vi "Control_Create.vi"(7 "Object Attributes":T1, 8 "error in (no error)":errorcluster, 10 "Control Attributes":T3, 11 "Control In":refnum<class "Control.lvclass">) -> (0 "error out":errorcluster, 3 "Control Out":refnum<class "Control.lvclass">)   [LabVIEW 2015, in "Front Panel Publisher.lvlib" / "Control.lvclass"]
uses:
  Control.lvclass
  Attributes.ctl
  Text_class/Text.lvclass
  Object_class/Attributes.ctl
  Object_class/Coordinates.ctl
  Object_class/Object.lvclass
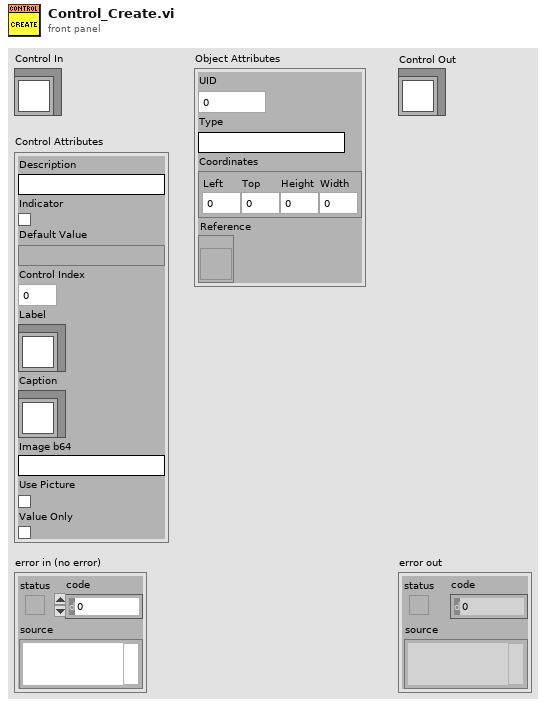
[diagram p1: front panel]
types:
  T1 = typedef "Front Panel Publisher.lvlib/Object.lvclass/Attributes.ctl" = cluster{"UID":i32, "Type":string, "Coordinates":T2, "Reference":refnum<vi>}
  T2 = typedef "Front Panel Publisher.lvlib/Object.lvclass/Coordinates.ctl" = cluster{"Left":i32, "Top":i32, "Height":u32, "Width":u32}
  T3 = typedef "Front Panel Publisher.lvlib/Control.lvclass/Attributes.ctl" = cluster{"Description":string, "Indicator":bool, "Default Value":variant, "Control Index":i32, "Label":refnum<class "Text.lvclass">, "Caption":refnum<class "Text.lvclass">, "Image b64":string, "Use Picture":bool, "Value Only":bool}
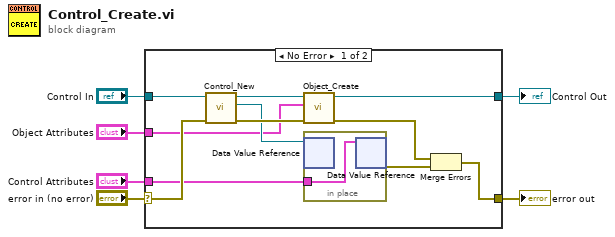
[diagram p0: block diagram]
diagram:
  n1 = case shown="No Error" "error in (no error)" {
    selector: "error in (no error)" -> [w16 w20]
    tunnel: [w14 w20] -> w5
    tunnel: "Control In" -> [w17 w19]
    tunnel: [w11 w19] -> w3
    tunnel: "Object Attributes" -> [w9 _]
    tunnel: "Control Attributes" -> [w8 _]
    frame No Error {
      n2 = call "Control_New.vi"("error in (no error)"=w16, "reference in"=w17) -> ("error out"=w12:errorcluster, "DVRRefOut"=w10:refnum<data-value>, "reference out"=w13:refnum<class "Control.lvclass">)  [unwired: 6 in, 1 out]
      n3 = call "Object_Create.vi"("error in (no error)"=w12, "Object Attributes"=w9, "Object In"=w13) -> ("error out"=w7:errorcluster, "Object Out"=w11:refnum<class "Control.lvclass">)  [unwired: 7 in]
      n4 = in-place {
        in-place-border: w8 -> [w18]
        n5 = in-place-dvr #1(w10) -> ()  [unwired: 2 out]
        n6 = in-place-dvr #1(w18) -> (w15:errorcluster)  [unwired: 1 out]
      }
      n7 = Merge Errors(w7, w15) -> (w14:errorcluster)
    }
    frame Error {
    }
  }
  "error out" <- w5
  "Control Out" <- w3
